vi "Process.vi"(8 "error in":errorcluster, 11 "Plugin in":refnum<class "MP710995.lvclass">) -> (0 "error out":errorcluster, 3 "Plugin out":refnum<class "MP710995.lvclass">)   [LabVIEW 2025, in "MP710995.lvlib" / "MP710995.lvclass"]
uses:
  MP710995.lvclass
  MP710995.lvclass/MP710995.ctl
  <vilib>/FlexLogger/SDK/PluginSDK.lvlibp/PEFClasses/SDK/Channel/ParameterAccess/Read DBL.vi
  <vilib>/FlexLogger/SDK/PluginSDK.lvlibp/PEFClasses/SDK/Plugin/Plugin.lvclass
  <vilib>/FlexLogger/SDK/PluginSDK.lvlibp/PEFClasses/SDK/Channel/Channel.lvclass
  C:/Program Files/National Instruments/LabVIEW 2025/vi.lib/FlexLogger/SDK/PluginSDK.lvlibp/PEFClasses/SDK/Plugin/Plugin.lvclass
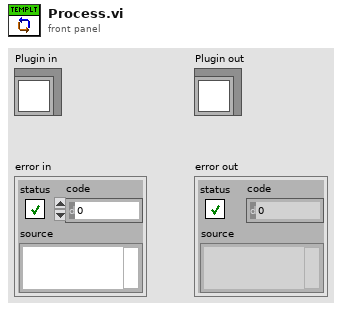
[diagram p1: front panel]
types:
  T1 = cluster{"Output":bool, "Current Limit":dbl, "Voltage":dbl, "Measured Voltage":dbl, "Measured Current":dbl, "OCP":bool}[]
  T2 = cluster{"Output":bool, "Current Limit":dbl, "Voltage":dbl, "Measured Voltage":dbl, "Measured Current":dbl, "OCP":bool}
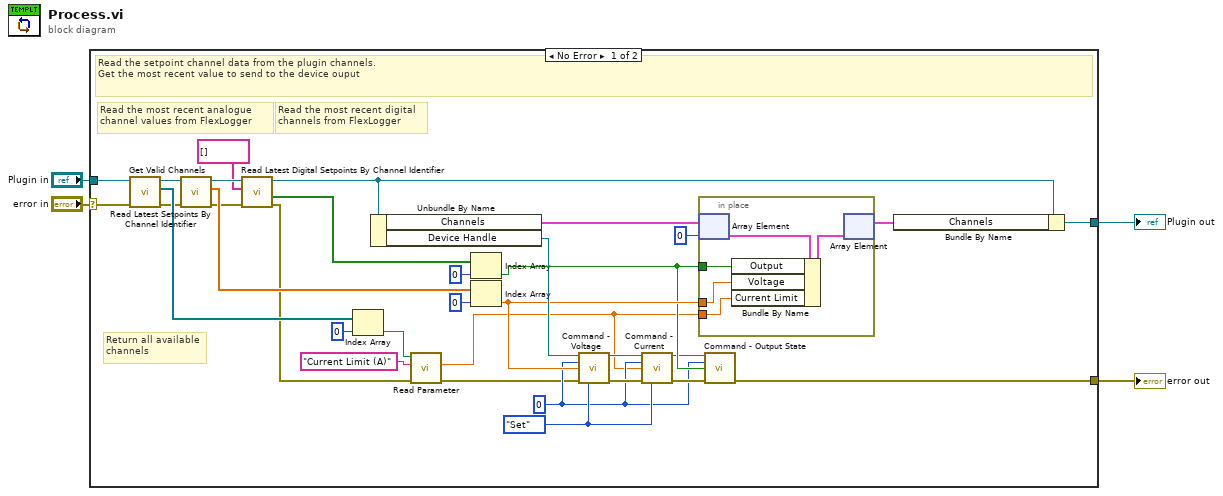
[diagram p0: block diagram]
diagram:
  n1 = case shown="No Error" "error in" {
    selector: "error in" -> [w13 w43]
    tunnel: [w37 w44] -> w4
    tunnel: "Plugin in" -> [w14 w44]
    tunnel: [w18 w43] -> w1
    frame No Error {
      w27 = enum16{"Set", "Get"}."Set" ("Command Type")
      w17 = 0 ("Channel")
      # "Return all available\nchannels"
      # "Read the most recent digital\nchannels from FlexLogger"
      # "Read the most recent analogue channel values from FlexLogger"
      # "Read the setpoint channel data from the plugin channels.\nGet the most recent value to send to the device ouput"
      n2 = call <vilib>:"Get Valid Channels.vi"("error in (no error)"=w13, "Plugin in"=w14) -> ("error out"=w8:errorcluster, "Channels"=w12:refnum<class "Channel.lvclass">[], "Plugin out"=w9:refnum<class "MP710995.lvclass">)  [unwired: 7 in]
      n3 = call <vilib>:"Read Latest Setpoints By Channel Identifier.vi"("error in (no error)"=w8, "Plugin in"=w9) -> ("error out"=w29:errorcluster, "Channel Setpoints"=w31:dbl[], "Plugin out"=w34:refnum<class "MP710995.lvclass">)  [unwired: 6 in, 1 out]
      n4 = call <vilib>:"Read Latest Digital Setpoints By Channel Identifier.vi"("error in (no error)"=w29, "Unique Channel Identifers (empty = all)"=string[] [], "Plugin in"=w34) -> ("error out"=w6:errorcluster, "Values"=w32:bool[], "Plugin out"=w16:refnum<class "MP710995.lvclass">)  [unwired: 5 in, 1 out]
      n5 = Index Array(array=w12, index=0) -> (element=w11:refnum<class "Channel.lvclass">)
      n6 = Unbundle By Name(w16) -> ("Channels"=w30:T1, "Device Handle"=w28:refnum<visa-resource-name>)
      n7 = call-poly <vilib>:"Read Parameter.vi"("error in (no error)"=w6, "Name"="Current Limit (A)", "Channel in"=w11) -> ("error out"=w7:errorcluster, "Value"=w5:dbl)  [unwired: 5 in, 2 out]
      n8 = Index Array(array=w32, index=0) -> (element=w25:bool)
      n9 = Index Array(array=w31, index=0) -> (element=w26:dbl)
      n10 = call "Command - Voltage.vi"("VISA Refnum in"=w28, "Channel"=w17, "Voltage"=w26, "Error In"=w7, "Command Type"=w27) -> ("VISA Refnum out"=w24:refnum<visa-resource-name>, "Error Out"=w22:errorcluster)  [unwired: 7 in, 2 out]
      n11 = call "Command - Current.vi"("VISA Refnum in"=w24, "Channel"=w17, "Current"=w5, "Error In"=w22, "Command Type"=w27) -> ("VISA Refnum out"=w23:refnum<visa-resource-name>, "Error Out"=w21:errorcluster)  [unwired: 7 in, 2 out]
      n12 = in-place {
        in-place-border: w25 -> [w41]
        in-place-border: w26 -> [w40]
        in-place-border: w5 -> [w39]
        n13 = in-place-array #1(w30, 0) -> (w42:T2)
        n14 = Bundle By Name(cluster=w42, "Output"=w41, "Voltage"=w40, "Current Limit"=w39) -> (w38:T2)
        n15 = in-place-array #1(w38) -> (w20:T1)  [unwired: 1 out]
      }
      n16 = call "Command - Output State.vi"("VISA Refnum in"=w23, "Channel"=w17, "State"=w25, "Error In"=w21) -> ("Error Out"=w18:errorcluster)  [unwired: 10 in, 1 out]
      n17 = Bundle By Name(cluster=w16, "Channels"=w20) -> (w37:refnum<class "MP710995.lvclass">)
    }
    frame Error {
    }
  }
  "error out" <- w1
  "Plugin out" <- w4
